vi "Correct Answer.vi"(8 "error in (no error)":errorcluster, 11 "MC Prompt in":refnum<class "MC Prompt.lvclass">) -> (0 "error out":errorcluster, 3 "MC Prompt out":refnum<class "MC Prompt.lvclass">)   [LabVIEW 2023, in "MC Prompt.lvlib" / "MC Prompt.lvclass"]
uses:
  MC Prompt.lvclass
  C:/Program Files/National Instruments/LabVIEW 2024/vi.lib/ActorFramework/Actor/Actor.lvclass
  <vilib>/ActorFramework/Actor/Actor.lvclass/Actor.ctl
  MC Prompt.lvclass/MC Prompt.ctl
  Controller/Controller Messages/Answer Received Msg/Answer Received Msg.lvclass/Answer Received Msg.ctl
  <vilib>/ActorFramework/Message Enqueuer/Message Enqueuer.lvclass/Message Enqueuer.ctl
  <vilib>/ActorFramework/Message Enqueuer/Enqueue.vi
  Controller/Controller Messages/Answer Received Msg/Answer Received Msg.lvclass
  C:/Program Files/National Instruments/LabVIEW 2024/vi.lib/ActorFramework/Message/Message.lvclass
  <vilib>/ActorFramework/Message Priority Queue/Priority Enqueue.vi
  <vilib>/ActorFramework/Actor/Actor.lvclass
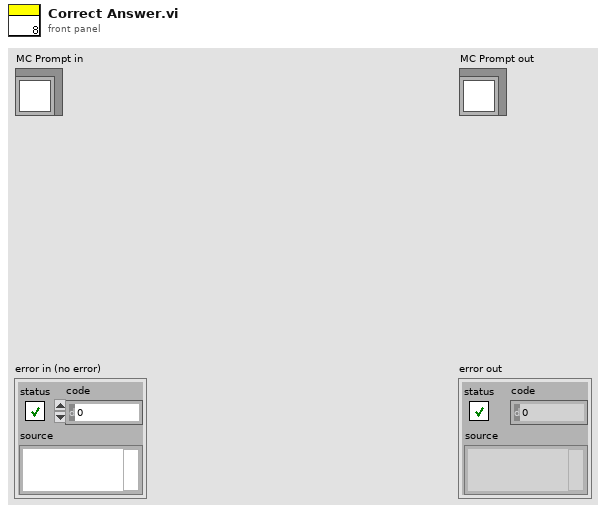
[diagram p1: front panel]
types:
  T1 = enum8{"Enabled", "Disabled", "Disabled and Grayed Out"}
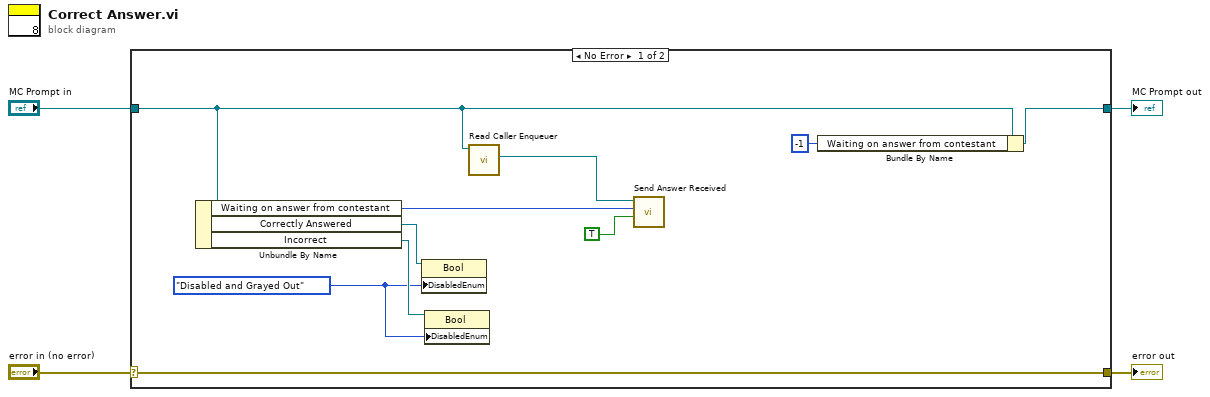
[diagram p0: block diagram]
diagram:
  n1 = case shown="No Error" "error in (no error)" {
    selector: "error in (no error)" -> [w14 w16]
    tunnel: [w14 w16] -> w3
    tunnel: [w13 w15] -> w1
    tunnel: "MC Prompt in" -> [w8 w15]
    frame No Error {
      w10 = T1."Disabled and Grayed Out" ("Disabled")
      n2 = Unbundle By Name(w8) -> ("Waiting on answer from contestant"=w6:i32, "Correctly Answered"=w12:refnum<vi>, "Incorrect"=w11:refnum<vi>)
      n3 = property class="Bool"(reference=w12, "DisabledEnum"=w10) -> ()  [unwired: 1 in, 2 out]
      n4 = property class="Bool"(reference=w11, "DisabledEnum"=w10) -> ()  [unwired: 1 in, 2 out]
      n5 = call <vilib>:"Read Caller Enqueuer.vi"("Actor"=w8) -> ("Caller Enqueuer"=w7:refnum<class "Message Enqueuer.lvclass">)  [unwired: 10 in]
      n6 = call "Send Answer Received.vi"("Correct?"=TRUE, "Contestant"=w6, "Message Enqueuer"=w7) -> ()  [unwired: 7 in, 2 out]
      n7 = Bundle By Name(cluster=w8, "Waiting on answer from contestant"=-1) -> (w13:refnum<class "MC Prompt.lvclass">)
    }
    frame Error {
    }
  }
  "error out" <- w3
  "MC Prompt out" <- w1
